vi "writeI24.vi"(8 "error in (no error)":errorcluster, 10 "Input":i32, 11 "ModbusBuffer in":refnum<class "ModbusBufferBuilder.lvclass">) -> (0 "error out":errorcluster, 3 "ModbusBuffer out":refnum<class "ModbusBufferBuilder.lvclass">)   [LabVIEW 2016, in "ModbusBufferBuilder.lvclass"]
uses:
  ModbusBufferBuilder.lvclass
  ModbusBufferBuilder.lvclass/ModbusBufferBuilder.ctl
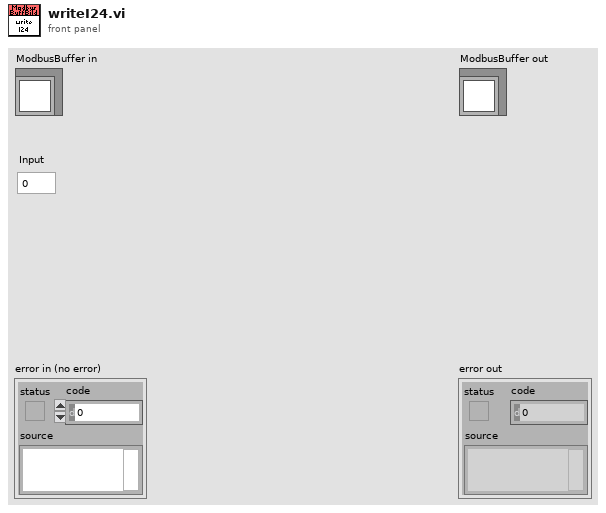
[diagram p1: front panel]
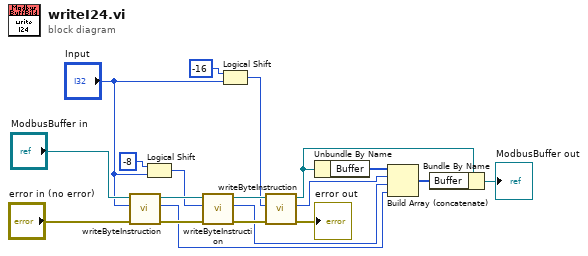
[diagram p0: block diagram]
diagram:
  n1 = call "writeByteInstruction.vi"("error in (no error)"="error in (no error)", "Input"="Input", "ModbusBuffer in"="ModbusBuffer in") -> ("error out"=w10:errorcluster, "Output"=w2:u16, "ModbusBuffer out"=w16:refnum<class "ModbusBufferBuilder.lvclass">)  [unwired: 6 in]
  n2 = Logical Shift(y=i16 -8, x="Input") -> (x << y=w13:i32)
  n3 = call "writeByteInstruction.vi"("error in (no error)"=w10, "Input"=w13, "ModbusBuffer in"=w16) -> ("error out"=w9:errorcluster, "Output"=w3:u16, "ModbusBuffer out"=w15:refnum<class "ModbusBufferBuilder.lvclass">)  [unwired: 6 in]
  n4 = Logical Shift(y=i16 -16, x="Input") -> (x << y=w12:i32)
  n5 = call "writeByteInstruction.vi"("error in (no error)"=w9, "Input"=w12, "ModbusBuffer in"=w15) -> ("error out"=→"error out":errorcluster, "Output"=w4:u16, "ModbusBuffer out"=w8:refnum<class "ModbusBufferBuilder.lvclass">)  [unwired: 6 in]
  n6 = Unbundle By Name(w8) -> ("Buffer"=w5:u16[])
  n7 = Build Array (concatenate)(w5, w4, w3, w2) -> (w1:u16[])
  n8 = Bundle By Name(cluster=w8, "Buffer"=w1) -> (→"ModbusBuffer out":refnum<class "ModbusBufferBuilder.lvclass">)
